vi "PSO_CalculateConstraints.vi"(8 "Fmax":i32, 10 "deltaF vector":i32[](array[numeric]), 11 "F0 vector":i32[](array[numeric])) -> (0 "Violation?":bool, 3 "Penalty":i32)   [LabVIEW 2016, in "Optimal Frequency Bands Search.lvlib" / "ParticleSwarm.lvlib"]
doc: "Рассчитать значение штрафной функции"
uses:
  ParticleSwarm.lvlib
panel:
  # "This VI is a part of BCI Design library, http://www.ru-bci.org \nCopyright © 2020, Sotnikov Peter, All rights reserved. License: GNU GPLv3"
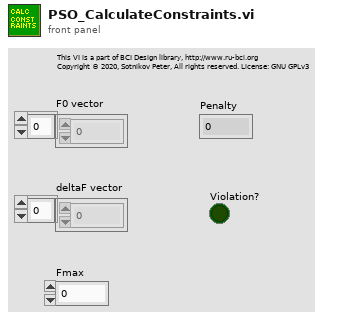
[diagram p1: front panel]
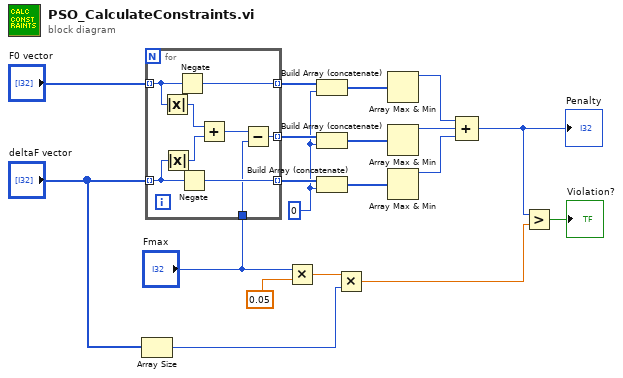
[diagram p0: block diagram]
diagram:
  w16 = 0 ("f")
  n1 = Array Size(array="deltaF vector") -> (size(s)=w4:i32)
  n2 = for {
    tunnel: "F0 vector" -> [w23] mode=indexing
    tunnel: "deltaF vector" -> [w22] mode=indexing
    tunnel: [w27] -> w19 mode=indexing
    tunnel: [w26] -> w18 mode=indexing
    tunnel: [w25] -> w17 mode=indexing
    tunnel: "Fmax" -> [w20]
    n3 = Absolute Value(x=w23) -> (abs(x)=w24:i32)
    n4 = Absolute Value(x=w22) -> (abs(x)=w21:i32)
    n5 = Negate(x=w23) -> (-x=w27:i32)
    n6 = Negate(x=w22) -> (-x=w25:i32)
    n7 = Add(x=w24, y=w21) -> (x+y=w28:i32)
    n8 = Subtract(x=w28, y=w20) -> (x-y=w26:i32)
  }
  n9 = Multiply(x="Fmax", y=0.05) -> (x*y=w6:dbl)
  n10 = Build Array (concatenate) "Build Array"(w19, w16) -> (w13:i32[])
  n11 = Build Array (concatenate)(w18, w16) -> (w14:i32[])
  n12 = Build Array (concatenate)(w17, w16) -> (w15:i32[])
  n13 = Multiply(x=w6, y=w4) -> (x*y=w3:dbl)
  n14 = Array Max & Min(array=w13) -> (max value=w12:i32)  [unwired: 3 out]
  n15 = Array Max & Min(array=w14) -> (max value=w11:i32)  [unwired: 3 out]
  n16 = Array Max & Min(array=w15) -> (max value=w10:i32)  [unwired: 3 out]
  n17 = Compound Arithmetic op=ADD(w12, w11, w10) -> (w2:i32)
  "Penalty" <- w2
  n18 = Greater?(x=w2, y=w3) -> (0:→"Violation?":bool)
